vi "Configure Trigger Slope [TS] Core.vi"(8 "error in (no error)":errorcluster, 10 "trigger slope (0: Positive)":i32(ring) items=["Positive", "Negative"], 11 "CS++DMM in":refnum<class "CS++DMM.lvclass">) -> (0 "error out":errorcluster, 3 "CS++DMM out":refnum<class "CS++DMM.lvclass">)   [LabVIEW 2013, in "CS++DMM.lvlib" / "CS++DMM.lvclass"]
doc: "This VI configures the polarity of the external trigger source of the DMM.\n\nNote:\n\n(1) This VI is part of the IviDmmTriggerSlope [TS] extension group."
uses:
  CS++DMM.lvclass
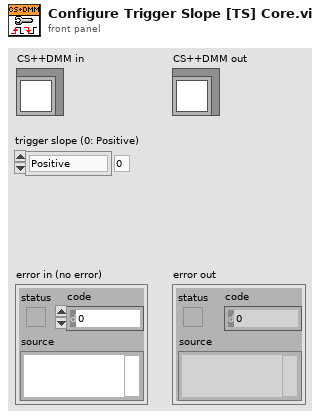
[diagram p1: front panel]
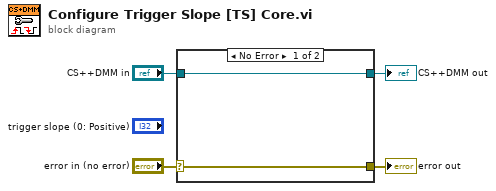
[diagram p0: block diagram]
diagram:
  n1 = case shown="No Error" "error in (no error)" {
    selector: "error in (no error)" -> [w5 w8]
    tunnel: [w5 w8] -> w3
    tunnel: [w6 w7] -> w1
    tunnel: "CS++DMM in" -> [w6 w7]
    frame No Error {
    }
    frame Error {
    }
  }
  "error out" <- w3
  "CS++DMM out" <- w1
